vi "DataTreeOrderSess.vi"(6 "Scans":cluster{i32[]}[](array[cluster]), 8 "error in (no error)":errorcluster, 9 "Scan":i32, 10 "Session":i32, 11 "SessTable":i32[](array[numeric])) -> (0 "error out":errorcluster, 2 "SessIndex":i32, 3 "SessTable Out":i32[](array[numeric]), 4 "Scans Out":cluster{i32[]}[](array[cluster]))   [LabVIEW 2019]
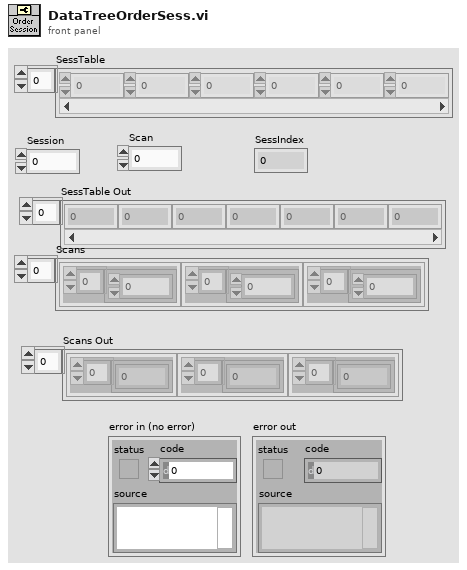
[diagram p1: front panel]
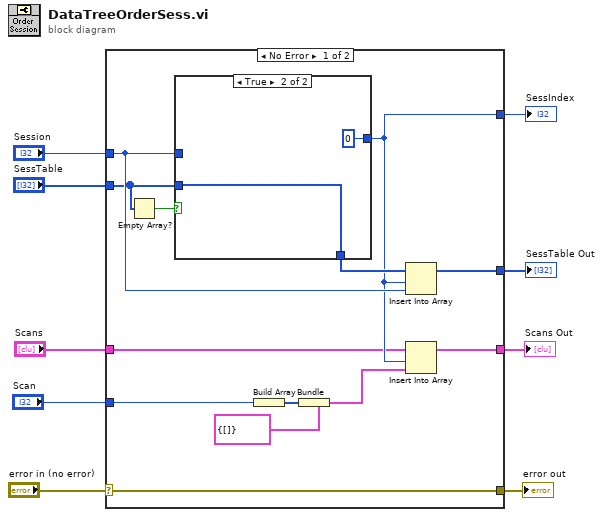
[diagram p0: block diagram]
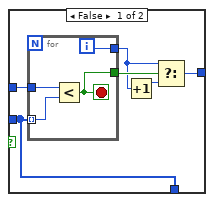
[diagram p2: hidden frame]
diagram:
  n1 = case shown="No Error" "error in (no error)" {
    selector: "error in (no error)" -> [w20 w35]
    tunnel: [w13 _] -> w9
    tunnel: "Session" -> [w22 _]
    tunnel: "SessTable" -> [w16 _]
    tunnel: [w21 _] -> w6
    tunnel: [w20 w35] -> w4
    tunnel: "Scan" -> [w19 _]
    tunnel: [w17 _] -> w2
    tunnel: "Scans" -> [w10 _]
    frame No Error {
      n2 = Empty Array?(array=w16) -> (empty?=w14:bool)
      n3 = case shown="True" w14 {
        tunnel: w22 -> [w28 _]
        tunnel: w16 -> [w23 w33]
        tunnel: [w24 0] -> w13
        tunnel: [w23 w33] -> w15
        frame False {
          n4 = for {
            tunnel: w23 -> [w31] mode=indexing
            tunnel: w28 -> [w32]
            tunnel: [w30] -> w25
            tunnel: [w29] -> w27
            i -> [w30]
            stop <- w29 stop-if-true
            n5 = Less?(x=w32, y=w31) -> (x < y?=w29:bool)
          }
          n6 = Increment(x=w25) -> (x+1=w26:i32)
          n7 = Select(t=w25, s=w27, f=w26) -> (s? t:f=w24:i32)
        }
        frame True {
        }
      }
      n8 = Build Array(w19) -> (w11:i32[])
      n9 = Bundle(cluster=cluster{i32[]} {[]} ("nouvel élément/sous-tableau"), w11) -> (w18:cluster{i32[]})
      n10 = Insert Into Array(array=w15, index=w13, new element=w22) -> (w21:i32[])
      n11 = Insert Into Array(array=w10, index=w13, new element=w18) -> (w17:cluster{i32[]}[])
    }
    frame Error {
    }
  }
  "SessIndex" <- w9
  "SessTable Out" <- w6
  "error out" <- w4
  "Scans Out" <- w2
